vi "GetVarVal_Array.vi"(8 "error in (no error)":errorcluster, 10 "varName":string, 11 "muExpr in":refnum<class "mupExpr.lvclass">) -> (0 "error out":errorcluster, 2 "varValue":dbl[](array[numeric]), 3 "muExpr out":refnum<class "mupExpr.lvclass">)   [LabVIEW 2018, in "mupExpr.lvclass"]
uses:
  mupExpr.lvclass
  mupExpr.lvclass/mupExpr.ctl
  <vilib>/Utility/error.llb/Error Cluster From Error Code.vi
  <vilib>/ErrorRing/Error Ring.xnode
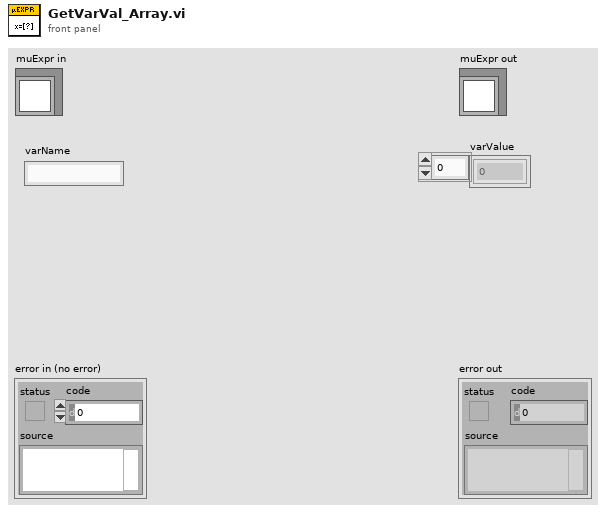
[diagram p1: front panel]
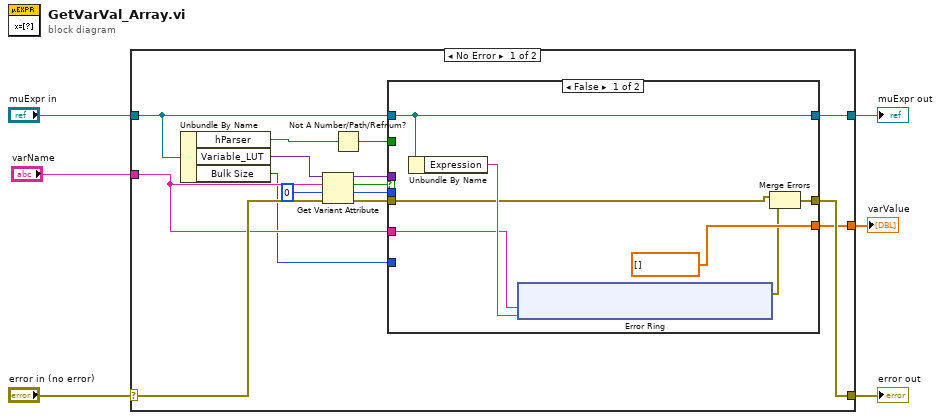
[diagram p0: block diagram]
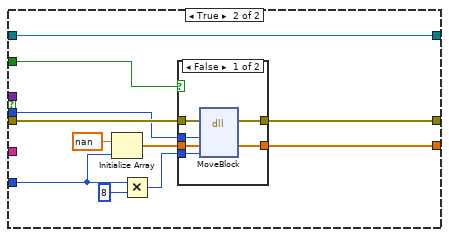
[diagram p2: hidden frame]
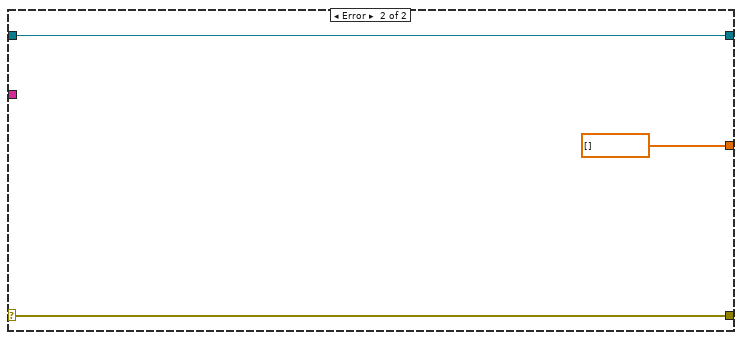
[diagram p4: hidden frame]
diagram:
  n1 = case shown="No Error" "error in (no error)" {
    selector: "error in (no error)" -> [w17 w58]
    tunnel: [w16 w58] -> w5
    tunnel: [w11 w57] -> w3
    tunnel: "muExpr in" -> [w13 w57]
    tunnel: "varName" -> [w14 _]
    tunnel: [w10 dbl[] [] ("varValue")] -> w1
    frame No Error {
      n2 = Unbundle By Name(w13) -> ("hParser"=w8:refnum<data-value>, "Variable_LUT"=w21:variant, "Bulk Size"=w9:i32)
      n3 = Get Variant Attribute(Variant=w21, name=w14, default value (empty Variant)=u64 0 ("pd"), error in=w17) -> (duplicate Variant=w12:variant, found=w15:bool, value=w18:u64, error out=w20:errorcluster)
      n4 = Not A Number/Path/Refnum?(number/path/refnum=w8) -> (NaN/Path/Refnum?=w7:bool)
      n5 = case shown="False" w15 {
        tunnel: w20 -> [w22 w46]
        tunnel: w18 -> [_ w44]
        tunnel: [w24 w45] -> w16
        tunnel: w14 -> [w25 _]
        tunnel: w13 -> [w28 w47]
        tunnel: w12 -> [_ _]
        tunnel: [w28 w47] -> w11
        tunnel: [dbl[] [] ("varValue") w43] -> w10
        tunnel: w9 -> [_ w39]
        tunnel: w7 -> [_ w37]
        frame False {
          n6 = Unbundle By Name(w28) -> ("Expression"=w26:string)
          n7 = xnode "Error Ring"("parameter 0"=w25, "parameter 1"=w26) -> ("error out"=w23:errorcluster)
          n8 = Merge Errors(w22, w23) -> (w24:errorcluster)
        }
        frame True {
          n9 = Initialize Array(nan ("element"), w39) -> (w40:dbl[])
          n10 = Multiply(x=w39, y=8) -> (x*y=w38:i32)
          n11 = case shown="False" w37 {
            tunnel: w46 -> [w53 w55]
            tunnel: [w52 w55] -> w45
            tunnel: w44 -> [w51 _]
            tunnel: [w50 w54] -> w43
            tunnel: w40 -> [w49 w54]
            tunnel: w38 -> [w48 _]
            frame False {
              n12 = dll-call lib="LabVIEW" fn="MoveBlock"(error in=w53, "ps"=w51, "pd"=w49, "size"=w48) -> (error out=w52:errorcluster, "pd"=w50:dbl[])  [unwired: 5 in, 1 out]
            }
            frame True {
            }
          }
        }
      }
    }
    frame Error {
    }
  }
  "error out" <- w5
  "muExpr out" <- w3
  "varValue" <- w1
